vi "FlatToRichni_measurementlink_PinMapContext.vi"(5 "OutputClusterType":T1, 11 "InputCluster":T2) -> (3 "OutputCluster":T1)   [LabVIEW 2020, in "MeasurementLink Measurement Service Base V2.lvlib"]
uses:
  MeasurementLink Measurement Service Base V2.lvlib
  ni_measurementlink_PinMapContext_Flat.ctl
  ni_measurementlink_PinMapContext.ctl
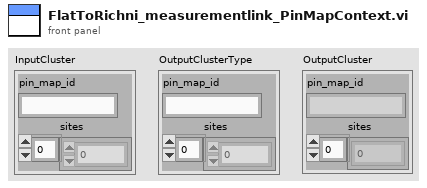
[diagram p1: front panel]
types:
  T1 = typedef "MeasurementLink Measurement Service Base V2.lvlib/ni_measurementlink_PinMapContext.ctl" = cluster{"pin_map_id":string, "sites":i32[]}
  T2 = typedef "MeasurementLink Measurement Service Base V2.lvlib/ni_measurementlink_PinMapContext_Flat.ctl" = cluster{"pin_map_id":string, "sites":i32[]}
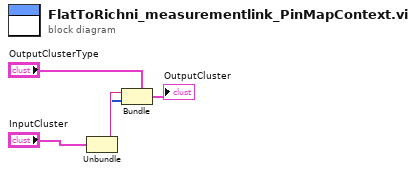
[diagram p0: block diagram]
diagram:
  n1 = Unbundle "Unbundle"("InputCluster") -> ("pin_map_id"=w2:string, "sites"=w1:i32[])
  n2 = Bundle "Bundle"(cluster="OutputClusterType", "pin_map_id"=w2, "sites"=w1) -> (→"OutputCluster":T1)
